vi "LVClass_HasoEngine Get Pixels Start Multi Aperture.vi"(0 "HasoEngine in":refnum<class "HasoEngine.lvclass">, 11 "error in (no error)":errorcluster) -> (4 "HasoEngine out":refnum<class "HasoEngine.lvclass">, 6 "Array":T1[](array[typedef]), 15 "error out":errorcluster)   [LabVIEW 2020, in "HasoEngine.lvclass"]
doc: "Get the shift values (in x and y direction) to apply to pair the start sub-\npupil with the appropriate micro-lens.\n\n--------------------------------------------------------------------------------\n\n<B>HasoEngineIn </B> : HasoEngine object.\n<B>HasoEngineOut </B> : HasoEngine object.\n<B>shift </B> : Alignment shift.\n<B>ErrorIn </B> : Error\n<B>ErrorOut </B> : Error\n\n--------------------------------------------------------------------------------"
uses:
  HasoEngine.lvclass
  Point2D.ctl
  HasoEngine.lvclass/HasoEngine.ctl
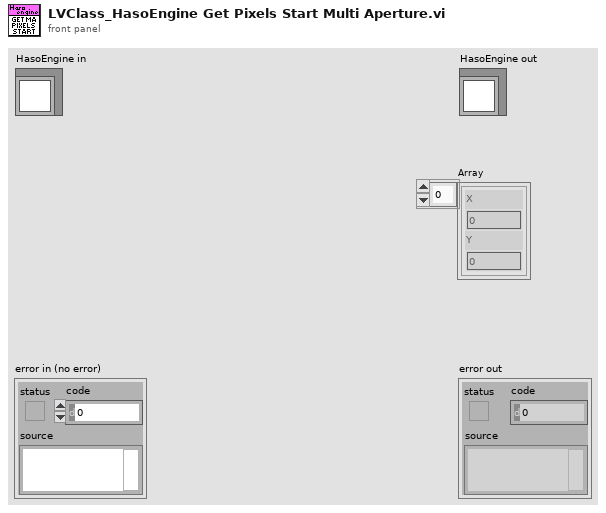
[diagram p1: front panel]
types:
  T1 = typedef "Point2D.ctl" = cluster{"X":u32, "Y":u32}
  T2 = typedef "ClassID.ctl" = i64
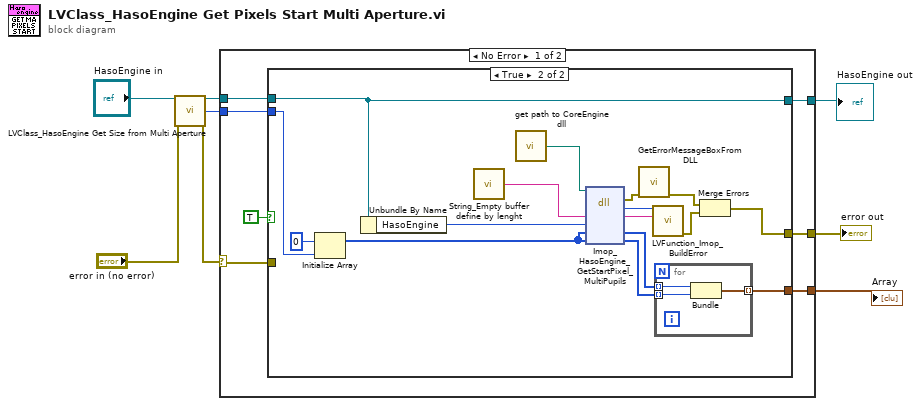
[diagram p0: block diagram]
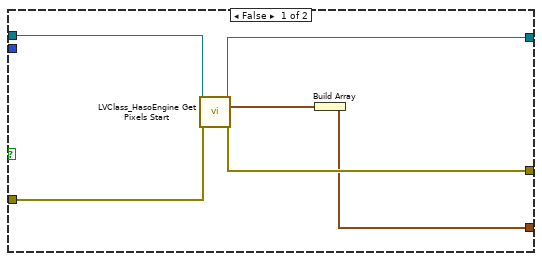
[diagram p2: hidden frame]
diagram:
  n1 = call "LVClass_HasoEngine Get Size from Multi Aperture.vi"("HasoEngine in"="HasoEngine in", "error in (no error)"="error in (no error)") -> ("HasoEngine out"=w3:refnum<class "HasoEngine.lvclass">, "Size"=w2:i32, "error out"=w5:errorcluster)  [unwired: 11 in]
  n2 = case shown="No Error" w5 {
    selector: w5 -> [w11 w41]
    tunnel: w3 -> [w15 w42]
    tunnel: [w9 w42] -> w7
    tunnel: [w14 w41] -> w8
    tunnel: w2 -> [w13 _]
    tunnel: [w12 _] -> w1
    frame No Error {
      n3 = case shown="True" TRUE {
        tunnel: w15 -> [w21 w22]
        tunnel: [w18 w29] -> w14
        tunnel: w13 -> [_ w27]
        tunnel: [w16 w23] -> w12
        tunnel: w11 -> [w19 _]
        tunnel: [w20 w22] -> w9
        frame False {
          n4 = call "LVClass_HasoEngine Get Pixels Start.vi"("HasoEngine in"=w21, "error in (no error)"=w19) -> ("HasoEngine out"=w20:refnum<class "HasoEngine.lvclass">, "pixel_start"=w17:T1, "error out"=w18:errorcluster)  [unwired: 11 in]
          n5 = Build Array(w17) -> (w16:T1[])
        }
        frame True {
          n6 = Initialize Array(u32 0 ("X"), w27) -> (w26:u32[])
          n7 = Unbundle By Name(w22) -> ("HasoEngine"=w32:T2)
          n8 = call "String_Empty buffer define by lenght.vi"() -> ("Empty buffer"=w37:string)  [unwired: 1 in]
          n9 = call "get path to CoreEngine dll.vi"() -> ("path to wavekit library"=w34:path)  [unwired: 14 in, 1 out]
          n10 = dll-call lib="D:/soft/HASO_v3/SVN_trunk/ImOpCoreEngine4_LV2011/DLLs/c_interface_vc100.dll" fn="Imop_HasoEngine_GetStartPixel_MultiPupils"(path in=w34, "message"=w37, "objet"=w32, "ArrayOfStartSubPupil_X"=w26, "ArrayOfStartSubPupil_Y"=w26) -> (error out=w33:errorcluster, "return type"=w35:i32, "message"=w36:string, "ArrayOfStartSubPupil_X"=w25:u32[], "ArrayOfStartSubPupil_Y"=w24:u32[])  [unwired: 3 in, 1 out]
          n11 = call "GetErrorMessageBoxFromDLL.vi"("error IN"=w33) -> ("error OUT"=w31:errorcluster)  [unwired: 10 in]
          n12 = call "LVFunction_Imop_BuildError.vi"("code"=w35, "String to Prepend to source (\"\")"=w36) -> ("error out"=w30:errorcluster)  [unwired: 13 in]
          n13 = for {
            tunnel: w25 -> [w40] mode=indexing
            tunnel: w24 -> [w39] mode=indexing
            tunnel: [w38] -> w23 mode=indexing
            n14 = Bundle(w40, w39) -> (w38:cluster{u32, u32})  [unwired: 1 in]
          }
          n15 = Merge Errors(w31, w30) -> (w29:errorcluster)
        }
      }
    }
    frame Error {
    }
  }
  "error out" <- w8
  "HasoEngine out" <- w7
  "Array" <- w1
